vi "EnumerateElements.vi"(8 "error in (no error)":errorcluster, 10 "Qualified Name":string, 11 "ConfigManager.Text in":refnum<class "ConfigManager.Text.lvclass">) -> (0 "error out":errorcluster, 2 "keys":string[](array[string]), 3 "ConfigManager.Text out":refnum<class "ConfigManager.Text.lvclass">)   [LabVIEW 2013, in "CfgManager.Text.lvlib" / "ConfigManager.Text.lvclass"]
uses:
  ConfigManager.Text.lvclass
  ConfigManager.Text.lvclass/ConfigManager.Text.ctl
  <vilib>/LabVIEW Open Source Project/Unicity/Delimiter/Delimiter.lvclass
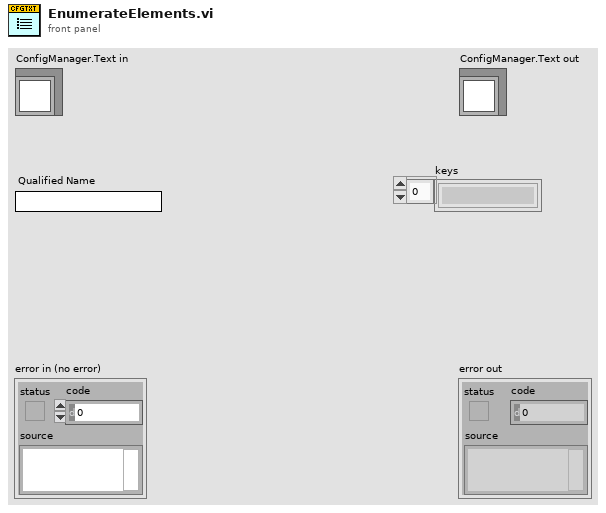
[diagram p1: front panel]
types:
  T1 = typedef "CfgManager.Text.lvlib/ConfigManager.Text.lvclass/Configuration -- Cluster.ctl" = cluster{"FileHeader":refnum<class "FileHeader.lvclass">, "FileSignature":refnum<class "FileSignature.lvclass">, "Section Delimiter":refnum<class "Delimiter.lvclass">, "Key-Value Separator":refnum<class "Delimiter.lvclass">}
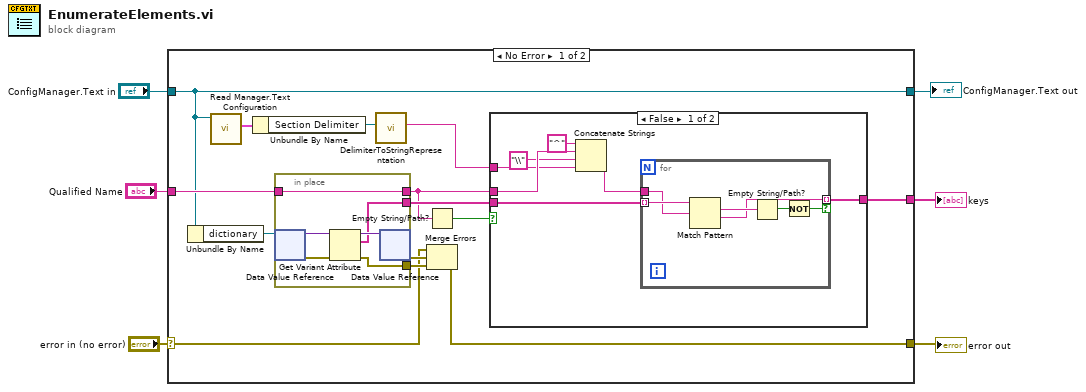
[diagram p0: block diagram]
diagram:
  n1 = case shown="No Error" "error in (no error)" {
    selector: "error in (no error)" -> [w16 w42]
    tunnel: [w20 w42] -> w1
    tunnel: "ConfigManager.Text in" -> [w8 w41]
    tunnel: [w8 w41] -> w5
    tunnel: [w11 _] -> w3
    tunnel: "Qualified Name" -> [w15 _]
    frame No Error {
      n2 = Unbundle By Name(w8) -> ("dictionary"=w17:refnum<data-value>)
      n3 = call "Read Manager.Text Configuration.vi"("ConfigManager.Text in"=w8) -> ("Manager.Text Configuration"=w9:T1)  [unwired: 9 in, 1 out]
      n4 = Unbundle By Name(w9) -> ("Section Delimiter"=w10:refnum<class "Delimiter.lvclass">)
      n5 = in-place {
        in-place-border: [w35] -> w19
        in-place-border: w15 -> [w36]
        in-place-border: [w37] -> w14
        in-place-border: [w36] -> w13
        n6 = in-place-dvr #1(w17) -> (w39:variant, w40:errorcluster)
        n7 = Get Variant Attribute(Variant=w39, error in=w40) -> (duplicate Variant=w38:variant, names=w37:string[], error out=w35:errorcluster)  [unwired: 2 in, 1 out]
        n8 = in-place-dvr #1(w38) -> (w18:errorcluster)  [unwired: 1 out]
      }
      n9 = call <vilib>:"DelimiterToStringRepresentation.vi"("Delimiter"=w10) -> ("String representation"=w7:string)  [unwired: 10 in]
      n10 = Empty String/Path?(string/path=w13) -> (empty?=w12:bool)
      n11 = Merge Errors(w16, w18, w19) -> (w20:errorcluster)
      n12 = case shown="False" w12 {
        tunnel: w14 -> [w27 w34]
        tunnel: w13 -> [w25 _]
        tunnel: [w26 w34] -> w11
        tunnel: w7 -> [w22 _]
        frame False {
          n13 = Concatenate Strings("^" ("string"), w25, "\\" ("string"), w22) -> (w24:string)
          n14 = for {
            tunnel: w24 -> [w29]
            tunnel: w27 -> [w31] mode=indexing
            tunnel: [w28] -> w26 mode=indexing if=w30
            n15 = Match Pattern(string=w31, regular expression=w29) -> (match substring=w33:string, after substring=w28:string)  [unwired: 1 in, 2 out]
            n16 = Empty String/Path?(string/path=w33) -> (empty?=w32:bool)
            n17 = Not(x=w32) -> (.not. x?=w30:bool)
          }
        }
        frame True {
        }
      }
    }
    frame Error {
    }
  }
  "error out" <- w1
  "ConfigManager.Text out" <- w5
  "keys" <- w3
